vi "get_cal_info.vi"(6 "timeout (25000ms)":i32=25000, 8 "error in (no error)":errorcluster, 10 "Mode":T2, 11 "daemon reference in":refnum<k5>) -> (0 "error out":errorcluster, 1 "Parameter":T1, 2 "response":string, 3 "daemon reference out":refnum<k5>, 5 "command out":string="random")   [LabVIEW 2017]
doc: "<b>Command: </b>\"get_cal_info\"\n\n<b>Description: </b> This command request device to read FCT/EOL/PROD calibration information. \n\n<b>Parameters: </b> Mode\n____________________________________________\nDIPC 692 Daemon API 10.0.0.1\nSam Tee - Dyson Technology Ltd\nCopyright (c) 2024, Dyson Technology Ltd"
uses:
  typdef/device_mode.ctl
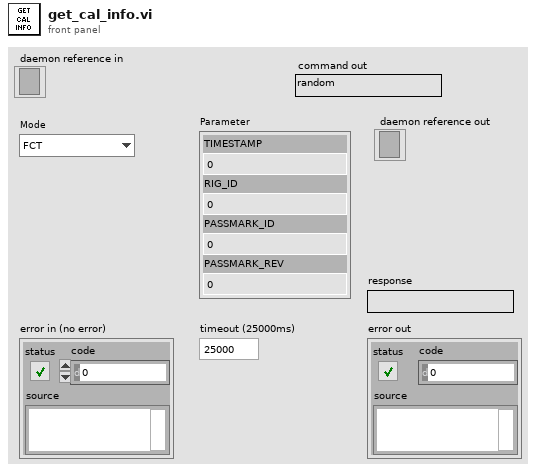
[diagram p1: front panel]
types:
  T1 = cluster{"TIMESTAMP":i64, "RIG_ID":i64, "PASSMARK_ID":i64, "PASSMARK_REV":i64}
  T2 = typedef "device_mode.ctl" = enum16{"FCT", "EOL", "PROD"}
  T3 = cluster{"[0]":i64, "[1]":i64, "[2]":i64, "[3]":i64}
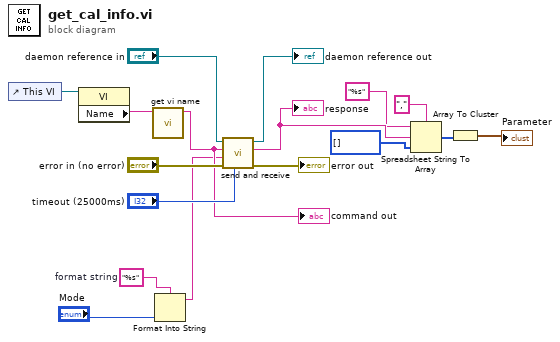
[diagram p0: block diagram]
diagram:
  w3 = "%s"  # format string
  n1 = control-ref of="This VI"() -> (w12:refnum<vi>)
  n2 = property class="VI"(reference=w12) -> ("Name"=w11:string)  [unwired: 1 in, 2 out]
  n3 = call "get vi name.vi"("library.lvlib:name.vi"=w11) -> ("vi name"=w10:string)  [unwired: 10 in]
  "command out" <- w10
  n4 = Format Into String(format string=w3, "Mode") -> (resulting string=w1:string)  [unwired: 2 in, 1 out]
  n5 = call "send and receive.vi"("timeout (25000ms)"="timeout (25000ms)", "error in (no error)"="error in (no error)", "data"=w1, "command"=w10, "daemon reference in"="daemon reference in") -> ("error out"=→"error out":errorcluster, "response"=w8:string, "daemon reference out"=→"daemon reference out":refnum<k5>)  [unwired: 4 in]
  "response" <- w8
  n6 = Spreadsheet String To Array(delimiter (Tab)=",", format string="%s", spreadsheet string=w8, array type (2D Dbl)=i64[] []) -> (array=w6:i64[])
  n7 = Array To Cluster(array=w6) -> (cluster=→"Parameter":T3)
